vi "Write Been Applied.vi"(8 "error in (no error)":errorcluster, 10 "Been Applied":bool, 11 "DriverSetting in":refnum<class "DriverSetting.lvclass">) -> (0 "error out":errorcluster, 3 "DriverSetting out":refnum<class "DriverSetting.lvclass">)   [LabVIEW 2023, in "HAF.lvlib" / "DriverSetting.lvclass"]
doc: "Saves an indication of whether or not the Driver Setting has been applied to the Instrument."
uses:
  DriverSetting.lvclass
  DriverSetting.lvclass/DriverSetting.ctl
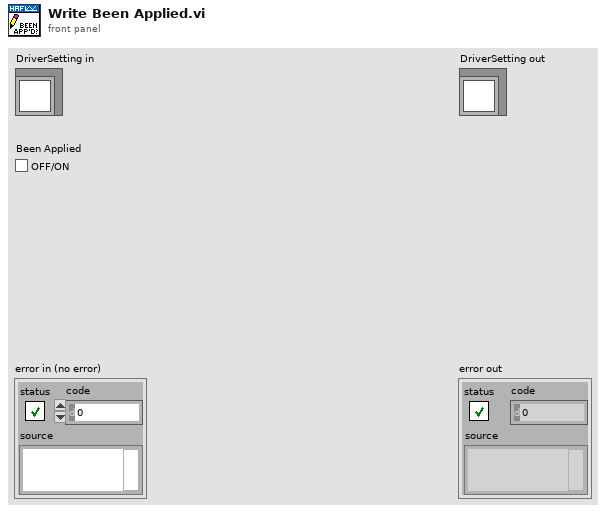
[diagram p1: front panel]
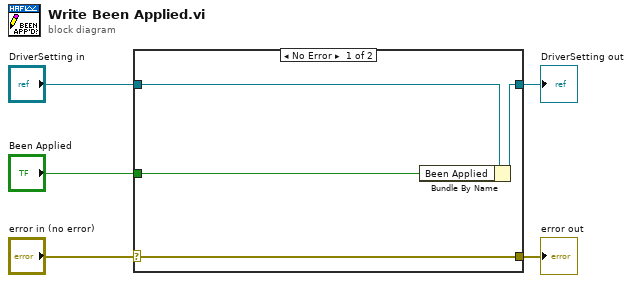
[diagram p0: block diagram]
diagram:
  n1 = case shown="No Error" "error in (no error)" {
    selector: "error in (no error)" -> [w9 w10]
    tunnel: [w9 w10] -> w4
    tunnel: [w7 w11] -> w2
    tunnel: "DriverSetting in" -> [w8 w11]
    tunnel: "Been Applied" -> [w6 _]
    frame No Error {
      n2 = Bundle By Name(cluster=w8, "Been Applied"=w6) -> (w7:refnum<class "DriverSetting.lvclass">)
    }
    frame Error {
    }
  }
  "error out" <- w4
  "DriverSetting out" <- w2
